vi "Ribbon Constructor.vi"(4 "Plot ID":i32, 6 "z matrix":sgl[][](array[numeric]), 8 "error in (no error)":errorcluster, 9 "y matrix":sgl[][](array[numeric]), 10 "x matrix":sgl[][](array[numeric]), 11 "3D Ribbon Datatype.lvclass in":refnum<class "3D Ribbon Datatype.lvclass">) -> (0 "error out":errorcluster, 3 "3D Ribbon Datatype.lvclass out":refnum<class "3D Ribbon Datatype.lvclass">)   [LabVIEW 2020, in "3D Ribbon Datatype.lvclass"]
uses:
  <vilib>/Math Plots/3D Math Plots/3D Ribbon/3D Ribbon Datatype/3D Ribbon Datatype.lvclass
  <vilib>/Math Plots/3D Math Plots/3D Ribbon/3D Ribbon Datatype/3D Ribbon Datatype.lvclass/3D Ribbon Datatype.ctl
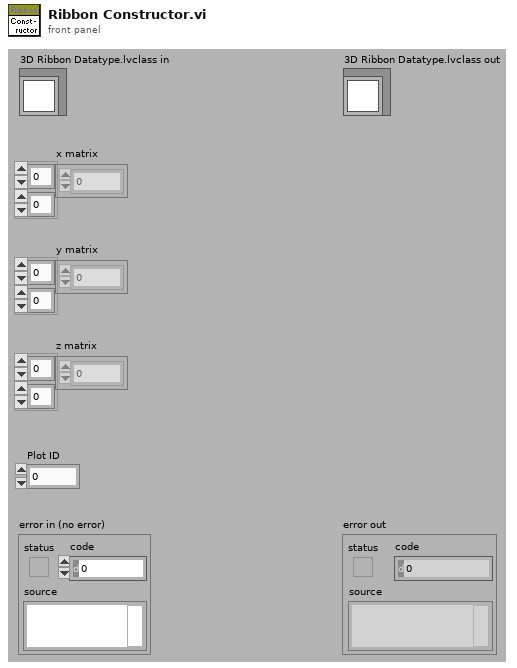
[diagram p1: front panel]
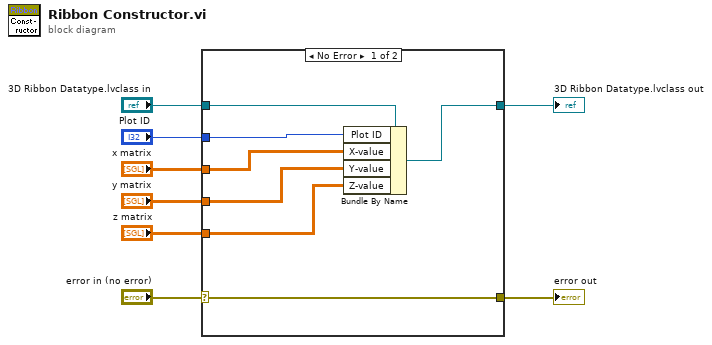
[diagram p0: block diagram]
diagram:
  n1 = case shown="No Error" "error in (no error)" {
    selector: "error in (no error)" -> [w13 w17]
    tunnel: "Plot ID" -> [w9 _]
    tunnel: [w13 w17] -> w7
    tunnel: "3D Ribbon Datatype.lvclass in" -> [w15 w16]
    tunnel: [w14 w16] -> w4
    tunnel: "x matrix" -> [w12 _]
    tunnel: "z matrix" -> [w11 _]
    tunnel: "y matrix" -> [w10 _]
    frame No Error {
      n2 = Bundle By Name(cluster=w15, "Plot ID"=w9, "X-value"=w12, "Y-value"=w10, "Z-value"=w11) -> (w14:refnum<class "3D Ribbon Datatype.lvclass">)
    }
    frame Error {
    }
  }
  "error out" <- w7
  "3D Ribbon Datatype.lvclass out" <- w4
